vi "Run.vi"(8 "error in (no error)":errorcluster, 11 "Project in":refnum<class "Job Initialize.lvclass">) -> (0 "error out":errorcluster, 2 "Text":string, 3 "Project out":refnum<class "Job Initialize.lvclass">)   [LabVIEW 2014, in "Job Initialize.lvclass"]
uses:
  Job Initialize.lvclass
  Job Initialize.lvclass/Job Initialize.ctl
  Build Job/Build Job.lvclass/Build Job.ctl
  Build Job/Read Parameters.vi
  Build Job/Write Parameters.vi
  Build Job/Build Job.lvclass
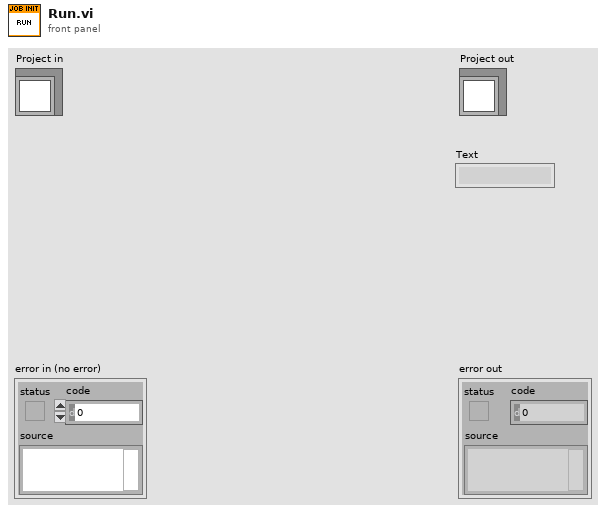
[diagram p1: front panel]
types:
  T1 = typedef "Source Code Control Selection - STYP.ctl" = enum16{"None (Manual Build)", "Every 15 Minutes", "Every 30 Minutes", "Every 45 Minutes", "Every Hour", "Every 2 Hours", "Everyday "}
  T2 = typedef "Cron String - STYP.ctl" = cluster{"Day of Week":enum16{"Everyday", "Sunday", "Monday", "Tuesday", "Wednesday", "Thursday", "Friday", "Saturday"}, "Hour":i32, "Enable?":bool}
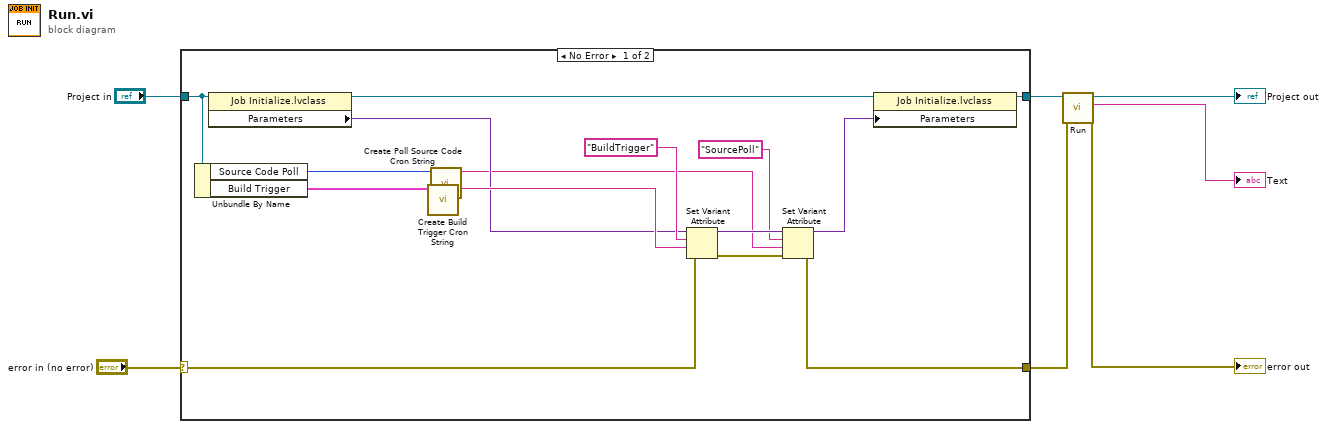
[diagram p0: block diagram]
diagram:
  n1 = case shown="No Error" "error in (no error)" {
    selector: "error in (no error)" -> [w10 w24]
    tunnel: [w14 w24] -> w1
    tunnel: [w22 w23] -> w3
    tunnel: "Project in" -> [w17 w23]
    frame No Error {
      n2 = Unbundle By Name(w17) -> ("Source Code Poll"=w9:T1, "Build Trigger"=w13:T2)
      n3 = property class="Job Initialize.lvclass"(reference=w17) -> (reference out=w16:refnum<class "Job Initialize.lvclass">, "Parameters"=w11:variant)  [unwired: 1 in, 1 out]
      n4 = call "Create Build Trigger Cron String.vi"("Cron"=w13) -> ("String"=w12:string)  [unwired: 10 in]
      n5 = call "Create Poll Source Code Cron String.vi"("Source Code Poll"=w9) -> ("String"=w8:string)  [unwired: 10 in]
      n6 = Set Variant Attribute(Variant=w11, name="BuildTrigger", value=w12, error in=w10) -> (Variant out=w20:variant, error out=w19:errorcluster)  [unwired: 1 out]
      n7 = Set Variant Attribute(Variant=w20, name="SourcePoll", value=w8, error in=w19) -> (Variant out=w15:variant, error out=w14:errorcluster)  [unwired: 1 out]
      n8 = property class="Job Initialize.lvclass"(reference=w16, "Parameters"=w15) -> (reference out=w22:refnum<class "Job Initialize.lvclass">)  [unwired: 1 in, 1 out]
    }
    frame Error {
    }
  }
  n9 = call-parent "Run.vi"("error in (no error)"=w1, "Project in"=w3) -> ("error out"=→"error out":errorcluster, "Text"=→"Text":string, "Project out"=→"Project out":refnum<class "Job Initialize.lvclass">)  [unwired: 7 in]
